vi "Pass.vi"(7 "Description":string, 8 "error in (no error)":errorcluster, 9 "Message":string, 11 "LUnit Test Case In":refnum<class "LUnit Test Case.lvclass">) -> (0 "error out":errorcluster, 3 "LUnit Test Case Out":refnum<class "LUnit Test Case.lvclass">)   [LabVIEW 2020, in "LUnit Test Case.lvclass"]
doc: "Generates a pass result for the calling test method. A description and message may be provided."
uses:
  LUnit Test Case.lvclass
  Result/Type.ctl
  LUnit Test Case.lvclass/LUnit Test Case.ctl
  Private/Run In UI.vi
  <vilib>/Utility/error.llb/Clear Errors.vi
  Result/Result.lvlib
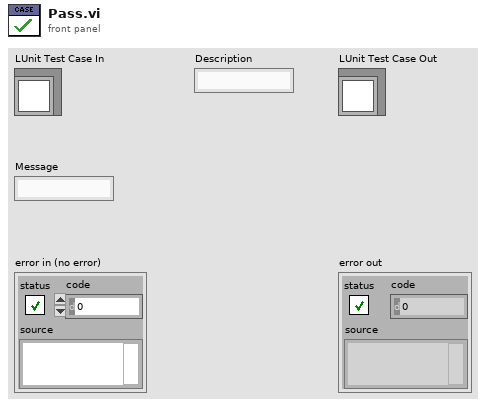
[diagram p1: front panel]
types:
  T1 = typedef "Result.lvlib/Type.ctl" = enum16{"Test Case", "Test Suite", "Test Run", "Pass", "Fail", "Skip", "Pass if", "Fail if", "Pass if Error", "Fail if Error", "Pass if Equal", "Fail if Equal"}
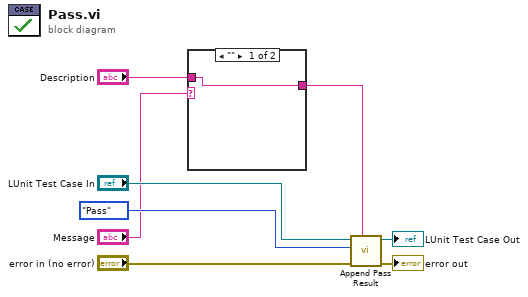
[diagram p0: block diagram]
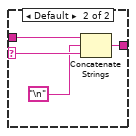
[diagram p2: hidden frame]
diagram:
  n1 = case shown="\"\"" "Message" {
    selector: "Message" -> [_ w11]
    tunnel: "Description" -> [w9 w13]
    tunnel: [w9 w12] -> w2
    frame "" {
    }
    frame Default {
      n2 = Concatenate Strings(w13, "\n", w11) -> (w12:string)
    }
  }
  n3 = call "Append Pass Result.vi"("Description"=w2, "error in (no error)"="error in (no error)", "Result Type"=Type."Pass", "LUnit Test Case In"="LUnit Test Case In") -> ("error out"=→"error out":errorcluster, "LUnit Test Case Out"=→"LUnit Test Case Out":refnum<class "LUnit Test Case.lvclass">)  [unwired: 6 in]
